vi "Config Parser.vi"(8 "error in (no error)":errorcluster, 10 "Config String":string, 11 "BML Pattern Creater in":refnum<class "BML Pattern Creater.lvclass">) -> (0 "error out":errorcluster, 3 "BML Pattern Creater out":refnum<class "BML Pattern Creater.lvclass">)   [LabVIEW 2018, in "BML Pattern Creater.lvlib" / "BML Pattern Creater.lvclass"]
uses:
  BML Pattern Creater.lvclass
  Ctls/FRM Data - BML.ctl
  Ctls/OM - BML.ctl
  Ctls/Burst Length.ctl
  Ctls/RW Options.ctl
  BML Pattern Creater.lvclass/BML Pattern Creater.ctl
  Write Frame Data.vi
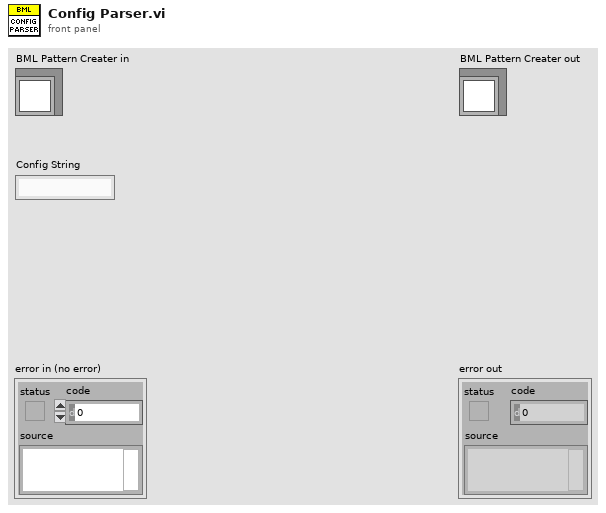
[diagram p1: front panel]
types:
  T1 = typedef "FRM Data - BML.ctl" = cluster{"Pattern_Name":string, "Data":u8[], "Start_Addr":u16, "ChipID":u8, "num of wait ms":i8, "Opcode":string[], "BML OM":T2, "BurstLength":T3, "FSN":u8, "R/W?":T4}
  T2 = typedef "OM - BML.ctl" = enum16{"Normal", "ImmeEffect", "InitSlaveID", "LoadData"}
  T3 = typedef "Burst Length.ctl" = enum8{"0", "2", "3", "4", "5", "8", "16", "32"}
  T4 = typedef "RW Options.ctl" = enum16{"Read", "Write", "R/W"}
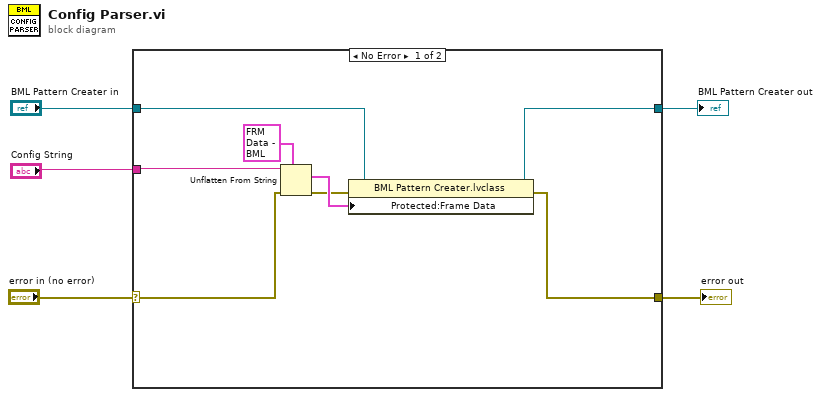
[diagram p0: block diagram]
diagram:
  n1 = case shown="No Error" "error in (no error)" {
    selector: "error in (no error)" -> [w12 w15]
    tunnel: [w10 w15] -> w4
    tunnel: [w11 w14] -> w2
    tunnel: "BML Pattern Creater in" -> [w13 w14]
    tunnel: "Config String" -> [w6 _]
    frame No Error {
      n2 = Unflatten From String(type=T1 {"Pattern_Name"="", "Data"=[], "Start_Addr"=0, "ChipID"=1, "num of wait ms"=0, "Opcode"=[], "BML OM"=enum."Normal", "BurstLength"=enum."0", "FSN"=0, "R/W?"=enum."Read"} ("Frame Data"), binary string=w6, error in (no error)=w12) -> (value=w8:T1, error out=w7:errorcluster)  [unwired: 2 in, 1 out]
      n3 = property class="BML Pattern Creater.lvclass"(reference=w13, error in=w7, "Protected:Frame Data"=w8) -> (reference out=w11:refnum<class "BML Pattern Creater.lvclass">, error out=w10:errorcluster)
    }
    frame Error {
    }
  }
  "error out" <- w4
  "BML Pattern Creater out" <- w2
